vi "DSF.Engine.Framework.Set Configuration.vi"(8 "error in (no error)":errorcluster, 10 "Framework Configuration":refnum<class "DSF.Shared.Configuration.Framework.lvclass">, 11 "Framework in":refnum<class "Framework.lvclass">) -> (0 "error out":errorcluster, 3 "Framework out":refnum<class "Framework.lvclass">)   [LabVIEW 2016, in "DSF.Engine.lvlib" / "Framework.lvclass"]
uses:
  Framework.lvclass
  Shared/Classes/Framework/DSF.Shared.Configuration.Framework.lvclass
  Framework.lvclass/Framework.ctl
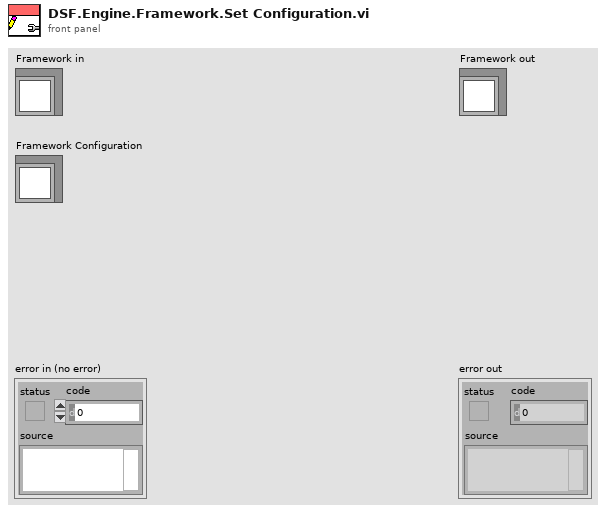
[diagram p1: front panel]
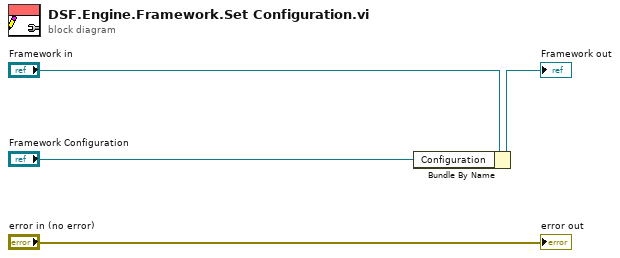
[diagram p0: block diagram]
diagram:
  n1 = Bundle By Name(cluster="Framework in", "Configuration"="Framework Configuration") -> (→"Framework out":refnum<class "Framework.lvclass">)
  "error out" <- "error in (no error)"
